vi "TestInitialOutput.vi"(10 "Delay Time (s)":dbl=0.4) -> (0 "Current output (mA)":dbl, 1 "Current (mA) level\nfor output pins":dbl[](array[numeric]), 2 "Delay Time":dbl)   [LabVIEW 2018]
uses:
  GlobalVariables/WaveformCharGlobal.vi
  <vilib>/express/express arith-compare/Formula/XNode/ExpressFormulaBlockNode.xnode
panel:
  in  "Fixed Resistor":dbl=350.0
  out "MUX channel":i32
  in  "stop":bool
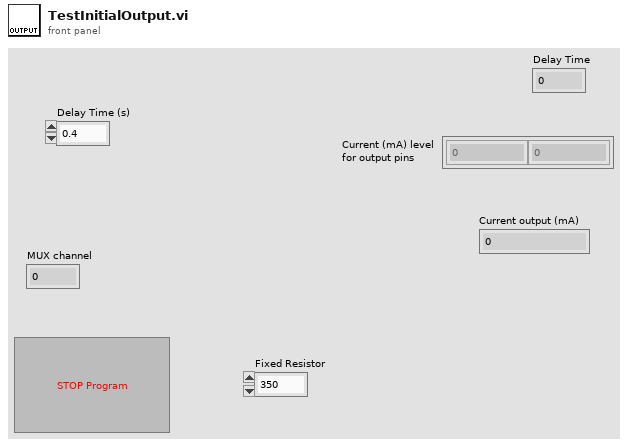
[diagram p1: front panel]
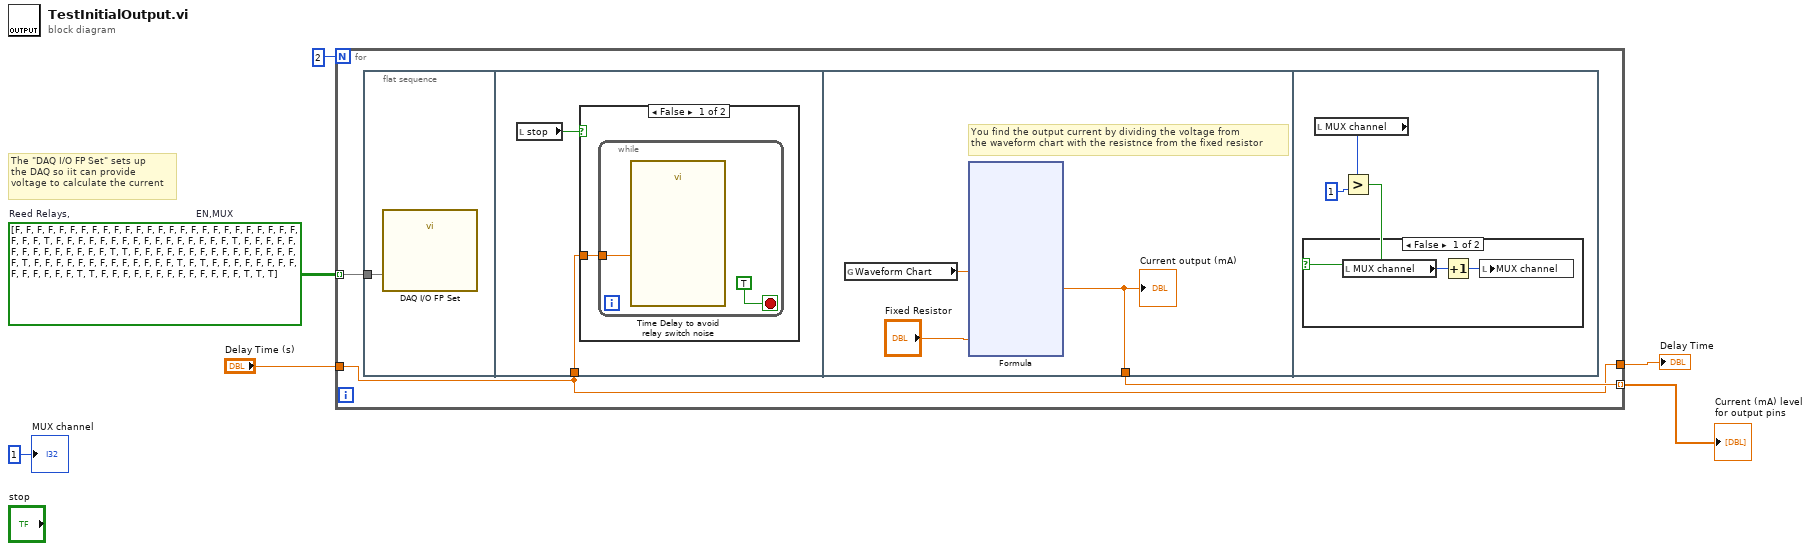
[diagram p0: block diagram]
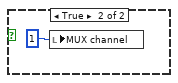
[diagram p3: hidden frame]
diagram:
  w5 = bool[][] [[FALSE, FALSE, FALSE, FALSE, FALSE, FALSE, FALSE, FALSE, FALSE, FALSE, FALSE, FALSE, FALSE, FALSE, FALSE, FALSE], [FALSE, FALSE, FALSE, FALSE, FALSE, FALSE, FALSE, FALSE, FALSE, FALSE, FALSE, FALSE, FALSE, TRUE, FALSE, FALSE], [FALSE, FALSE, FALSE, FALSE, FALSE, FALSE, FALSE, FALSE, FALSE, FALSE, FALSE, FALSE, FALSE, FALSE, TRUE, FALSE], [FALSE, FALSE, FALSE, FALSE, FALSE, FALSE, FALSE, FALSE, FALSE, FALSE, FALSE, FALSE, FALSE, TRUE, TRUE, FALSE], [FALSE, FALSE, FALSE, FALSE, FALSE, FALSE, FALSE, FALSE, FALSE, FALSE, FALSE, FALSE, FALSE, FALSE, FALSE, TRUE], [FALSE, FALSE, FALSE, FALSE, FALSE, FALSE, FALSE, FALSE, FALSE, FALSE, FALSE, FALSE, FALSE, TRUE, FALSE, TRUE], [FALSE, FALSE, FALSE, FALSE, FALSE, FALSE, FALSE, FALSE, FALSE, FALSE, FALSE, FALSE, FALSE, FALSE, TRUE, TRUE], [FALSE, FALSE, FALSE, FALSE, FALSE, FALSE, FALSE, FALSE, FALSE, FALSE, FALSE, FALSE, FALSE, TRUE, TRUE, TRUE]]  # Reed Relays,                                          EN,MUX
  # "The \"DAQ I/O FP Set\" sets up \nthe DAQ so iit can provide \nvoltage to calculate the current"
  n1 = for {
    N: 2 -> [_]
    tunnel: w5 -> [w9] mode=indexing
    tunnel: [w8] -> w6 mode=indexing
    tunnel: "Delay Time (s)" -> [w7]
    tunnel: [w7] -> w1
    n2 = flat-sequence {
      tunnel: w9 -> [w10]
      tunnel: w7 -> [w11]
      tunnel: [w16] -> w8
      frame #0 {
        n3 = call "DAQ I/O FP Set"("data"=w10) -> ()  [unwired: 17 in, 2 out]
      }
      frame #1 {
        n4 = local read "stop"() -> (w12:bool)
        n5 = case shown="False" w12 {
          tunnel: w11 -> [w13 _]
          frame False {
            n6 = while {
              tunnel: w13 -> [w14]
              stop <- TRUE stop-if-true
              n7 = call "Time Delay to avoid relay switch noise"("Delay Time (s)"=w14) -> ()  [unwired: 10 in, 1 out]
            }
          }
          frame True {
          }
        }
      }
      frame #2 {
        # "You find the output current by dividing the voltage from \nthe waveform chart with the resistnce from the fixed resistor"
        n8 = global read "WaveformCharGlobal.vi" "Waveform Chart"() -> (w17:dbl)
        n9 = xnode "Formula"("X1"=w17, "X2"="Fixed Resistor") -> ("Result"=w16:dbl)  [unwired: 1 in, 1 out]
        "Current output (mA)" <- w16
      }
      frame #3 {
        n10 = local read "MUX channel"() -> (w30:i32)
        n11 = Greater?(x=w30, y=1) -> (0:w31:bool)
        n12 = case shown="False" w31 {
          frame False {
            n13 = local read "MUX channel"() -> (w33:i32)
            n14 = Increment(x=w33) -> (x+1=w32:i32)
            n15 = local write "MUX channel"(w32) -> ()
          }
          frame True {
            n16 = local write "MUX channel"(1 ("MUX channel")) -> ()
          }
        }
      }
    }
  }
  "Current (mA) level\nfor output pins" <- w6
  "Delay Time" <- w1
  "MUX channel" <- 1 ("MUX channel")
